vi "setLaguerreOrder.vi"(8 "error in (no error)":errorcluster, 10 "LaguerreOrder":u32, 11 "LaguerreDeconClass in":refnum<class "LaguerreDeconEngineClass.lvclass">) -> (0 "error out":errorcluster, 3 "LaguerreDeconClass out":refnum<class "LaguerreDeconEngineClass.lvclass">)   [LabVIEW 2024, in "LaguerreDeconEngineClass.lvclass"]
uses:
  LaguerreDeconEngineClass.lvclass
  LaguerreDeconEngineClass.lvclass/LaguerreDeconEngineClass.ctl
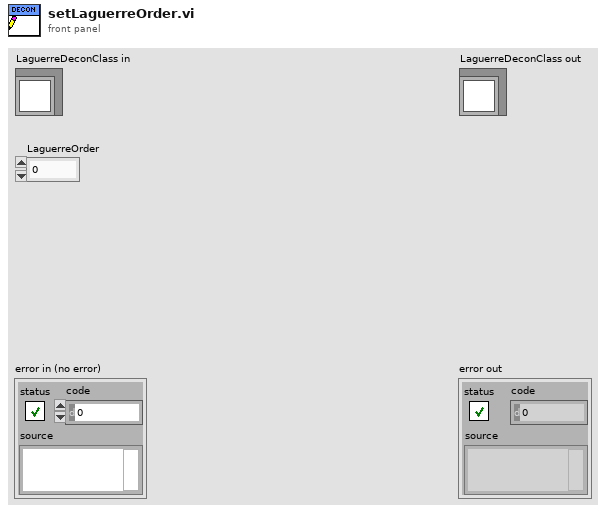
[diagram p1: front panel]
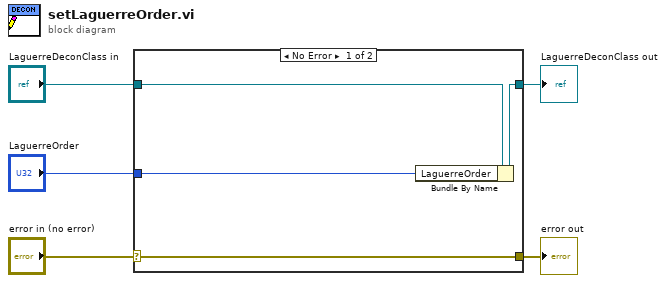
[diagram p0: block diagram]
diagram:
  n1 = case shown="No Error" "error in (no error)" {
    selector: "error in (no error)" -> [w9 w10]
    tunnel: [w9 w10] -> w4
    tunnel: [w7 w11] -> w2
    tunnel: "LaguerreDeconClass in" -> [w8 w11]
    tunnel: "LaguerreOrder" -> [w6 _]
    frame No Error {
      n2 = Bundle By Name(cluster=w8, "LaguerreOrder"=w6) -> (w7:refnum<class "LaguerreDeconEngineClass.lvclass">)
    }
    frame Error {
    }
  }
  "error out" <- w4
  "LaguerreDeconClass out" <- w2
